vi "AllMat_hyst_sat_concat.vi"(5 "N_sat":i32, 6 "AllMatrix":dbl[](array[numeric]), 7 "N_hyst":i32, 8 "sat_ds":T1, 9 "sat_ws":T1, 10 "r_s":T1, 11 "w_s":T1) -> (3 "Array":dbl[](array[numeric]))   [LabVIEW 2017]
uses:
  <vilib>/Analysis/Matrix/Datatypes/RealMatrix.ctl
  labview/utils_lib/utils.lvlib
  <vilib>/Analysis/Matrix/NI_Matrix.lvlib
panel:
  out "appended array":dbl[](array[numeric])
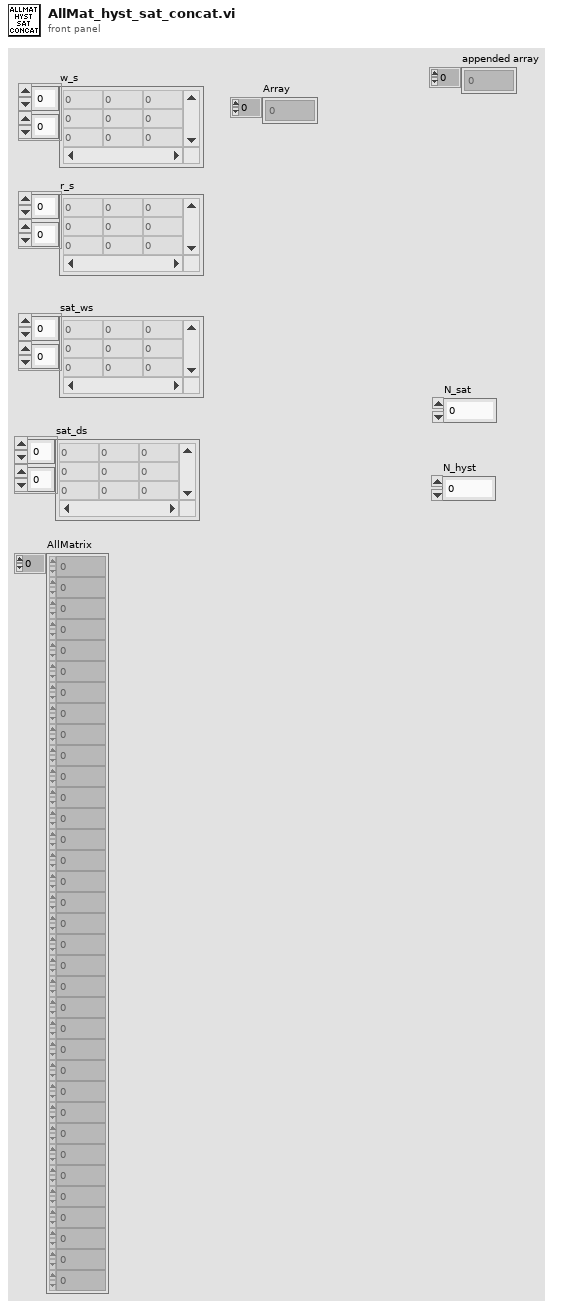
[diagram p1: front panel]
types:
  T1 = typedef "NI_Matrix.lvlib/RealMatrix.ctl" = dbl[][]
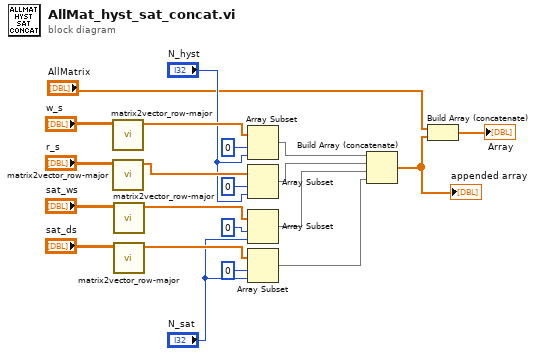
[diagram p0: block diagram]
diagram:
  n1 = call "matrix2vector_row-major.vi"("Matrix"="w_s") -> ("vector"=w21:dbl[])  [unwired: 10 in]
  n2 = call "matrix2vector_row-major.vi"("Matrix"="r_s") -> ("vector"=w20:dbl[])  [unwired: 10 in]
  n3 = call "matrix2vector_row-major.vi"("Matrix"="sat_ws") -> ("vector"=w10:dbl[])  [unwired: 10 in]
  n4 = call "matrix2vector_row-major.vi"("Matrix"="sat_ds") -> ("vector"=w9:dbl[])  [unwired: 10 in]
  n5 = Array Subset(array=w21, index=0, length="N_hyst") -> (w16:dbl[])
  n6 = Array Subset(array=w20, index=0, length="N_hyst") -> (w15:dbl[])
  n7 = Array Subset(array=w10, index=0, length="N_sat") -> (w12:dbl[])
  n8 = Array Subset(array=w9, index=0, length="N_sat") -> (w11:dbl[])
  n9 = Build Array (concatenate)(w16, w15, w12, w11) -> (w7:dbl[])
  "appended array" <- w7
  n10 = Build Array (concatenate)("AllMatrix", w7) -> (→"Array":dbl[])
